vi "string_to_array.vi"(10 "list state:arg":string) -> (2 "state:arg array":string[](array[string]))   [LabVIEW 2015]
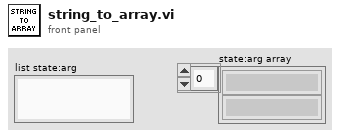
[diagram p1: front panel]
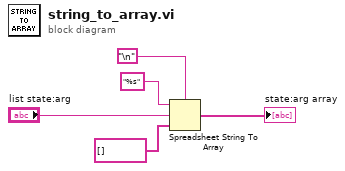
[diagram p0: block diagram]
diagram:
  n1 = Spreadsheet String To Array(delimiter (Tab)="\n", format string="%s", spreadsheet string="list state:arg", array type (2D Dbl)=string[] []) -> (array=→"state:arg array":string[])
